vi "altimeter decode.vi"(11 "string":string) -> (3 "before substring":string)   [LabVIEW 2021]
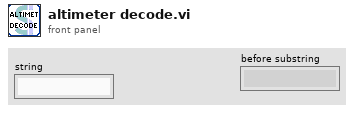
[diagram p1: front panel]
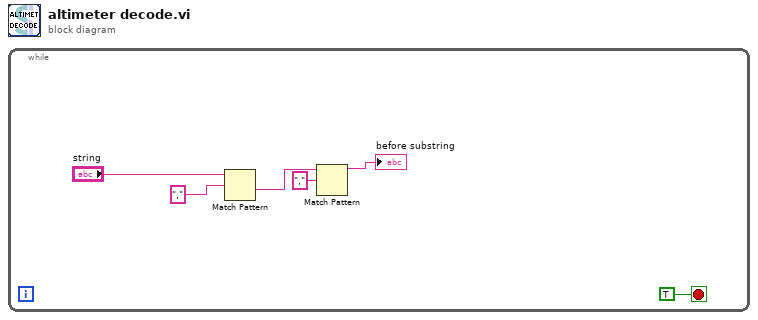
[diagram p0: block diagram]
diagram:
  n1 = while {
    stop <- TRUE stop-if-true
    n2 = Match Pattern(string="string", regular expression=",") -> (after substring=w4:string)  [unwired: 1 in, 3 out]
    n3 = Match Pattern(string=w4, regular expression=",") -> (before substring=→"before substring":string)  [unwired: 1 in, 3 out]
  }
